vi "pulse Tx 16 spc.vi"(8 "clear DDS":bool, 9 "enable line":bool=TRUE, 10 "take it!":bool, 11 "Cluster":T2={"PW"=0, "frequency shift"=0.0, "amp"=0.9999923706054688, "mode type"=enum."CW", "mode depth"=0, "mode filter"=0, "phase shift"=0.0, "pulse shape filter"=0}) -> (0 "output valid":bool, 1 "IQ out":T1[](array[typedef]), 2 "free dds":bool, 4 "frequncy":fxp<+/-,48,0>, 6 "phase":fxp<+/-,16,1>)   [LabVIEW 2021]
uses:
  pulse_tx_vis/pdw.ctl
  pulse_tx_vis/CTL/mode_type.ctl
  <instrlib>/_niInstr/DSP/v1/Shared/Public/IQ Data.ctl
  <instrlib>/_niInstr/DSP/v1/FPGA/Public/Sub VIs/Frequency Shift/Frequency Shift - 16 spc.vi
  <instrlib>/_niInstr/Basic Elements/v1/FPGA/Private/Count Up U32.vi
  <vilib>/rvi/FXPMathLib/FxpAdd/XNode/nifxpmath_Add.xnode
  <instrlib>/_niInstr/DSP/v1/Shared/niInstr DSP v1 Shared.lvlib
  <instrlib>/_niInstr/Basic Elements/v1/FPGA/niInstr Basic Elements v1 FPGA.lvlib
  <vilib>/rvi/FXPMathLib/sim/FxpSim.dll
  <instrlib>/_niInstr/DSP/v1/FPGA/niInstr DSP v1 FPGA.lvlib
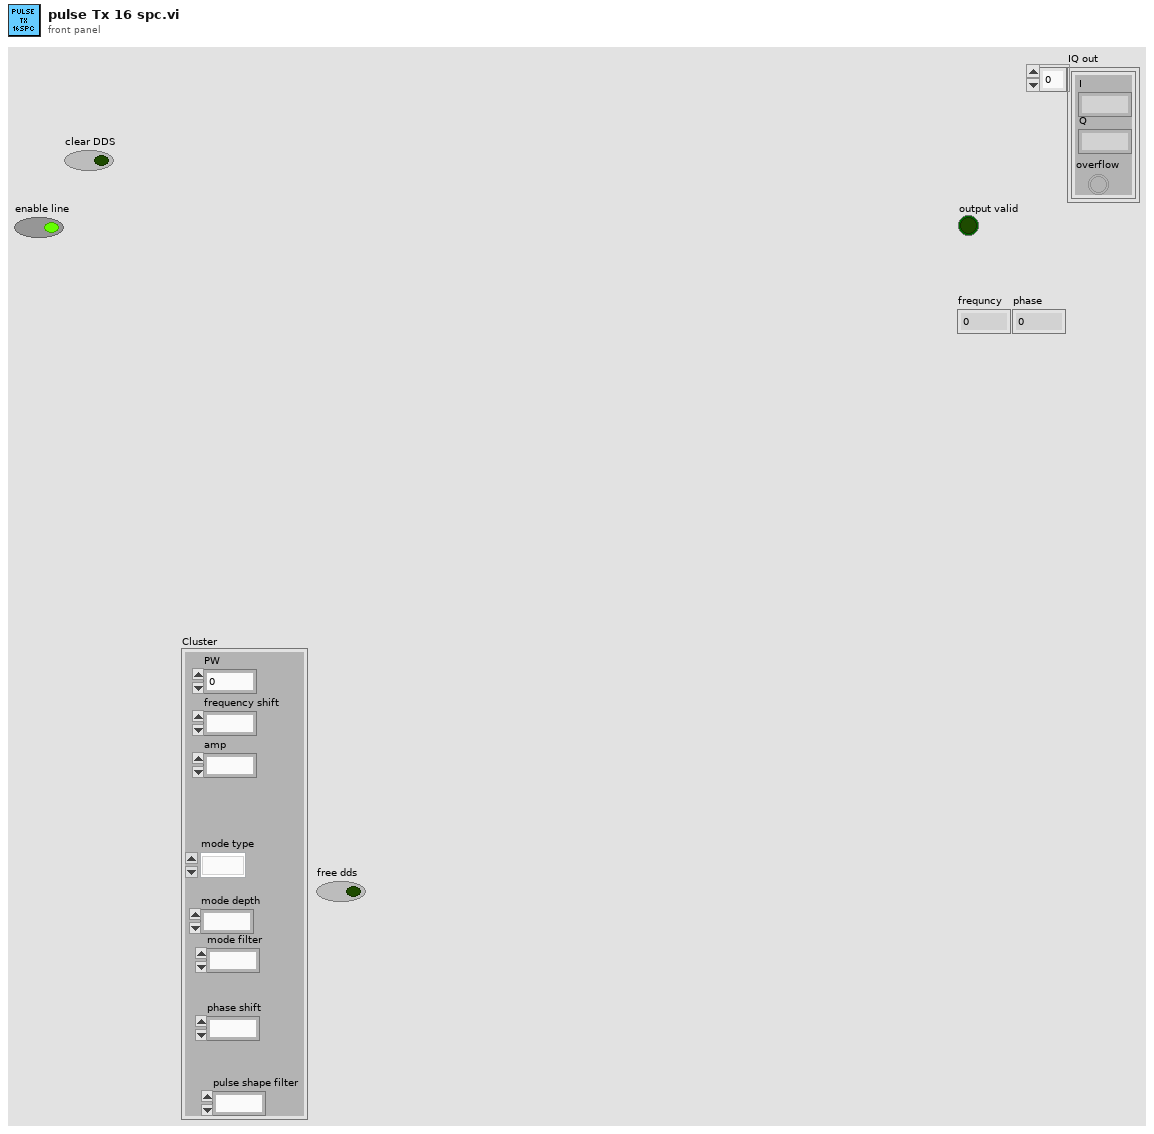
[diagram p1: front panel]
types:
  T1 = typedef "niInstr DSP v1 Shared.lvlib/IQ Data.ctl" = cluster{"I":fxp<+/-,18,1>, "Q":fxp<+/-,18,1>, "overflow":bool}
  T2 = typedef "pdw.ctl" = cluster{"PW":u32, "frequency shift":fxp<+/-,48,0>, "amp":fxp<+/-,18,1>, "mode type":T3, "mode depth":u32, "mode filter":u8, "phase shift":fxp<+/-,16,1>, "pulse shape filter":u8}
  T3 = typedef "mode_type.ctl" = enum8{"CW", "from memory 1", "NC - cw", "LFM", "BPSK", "QPSK"}
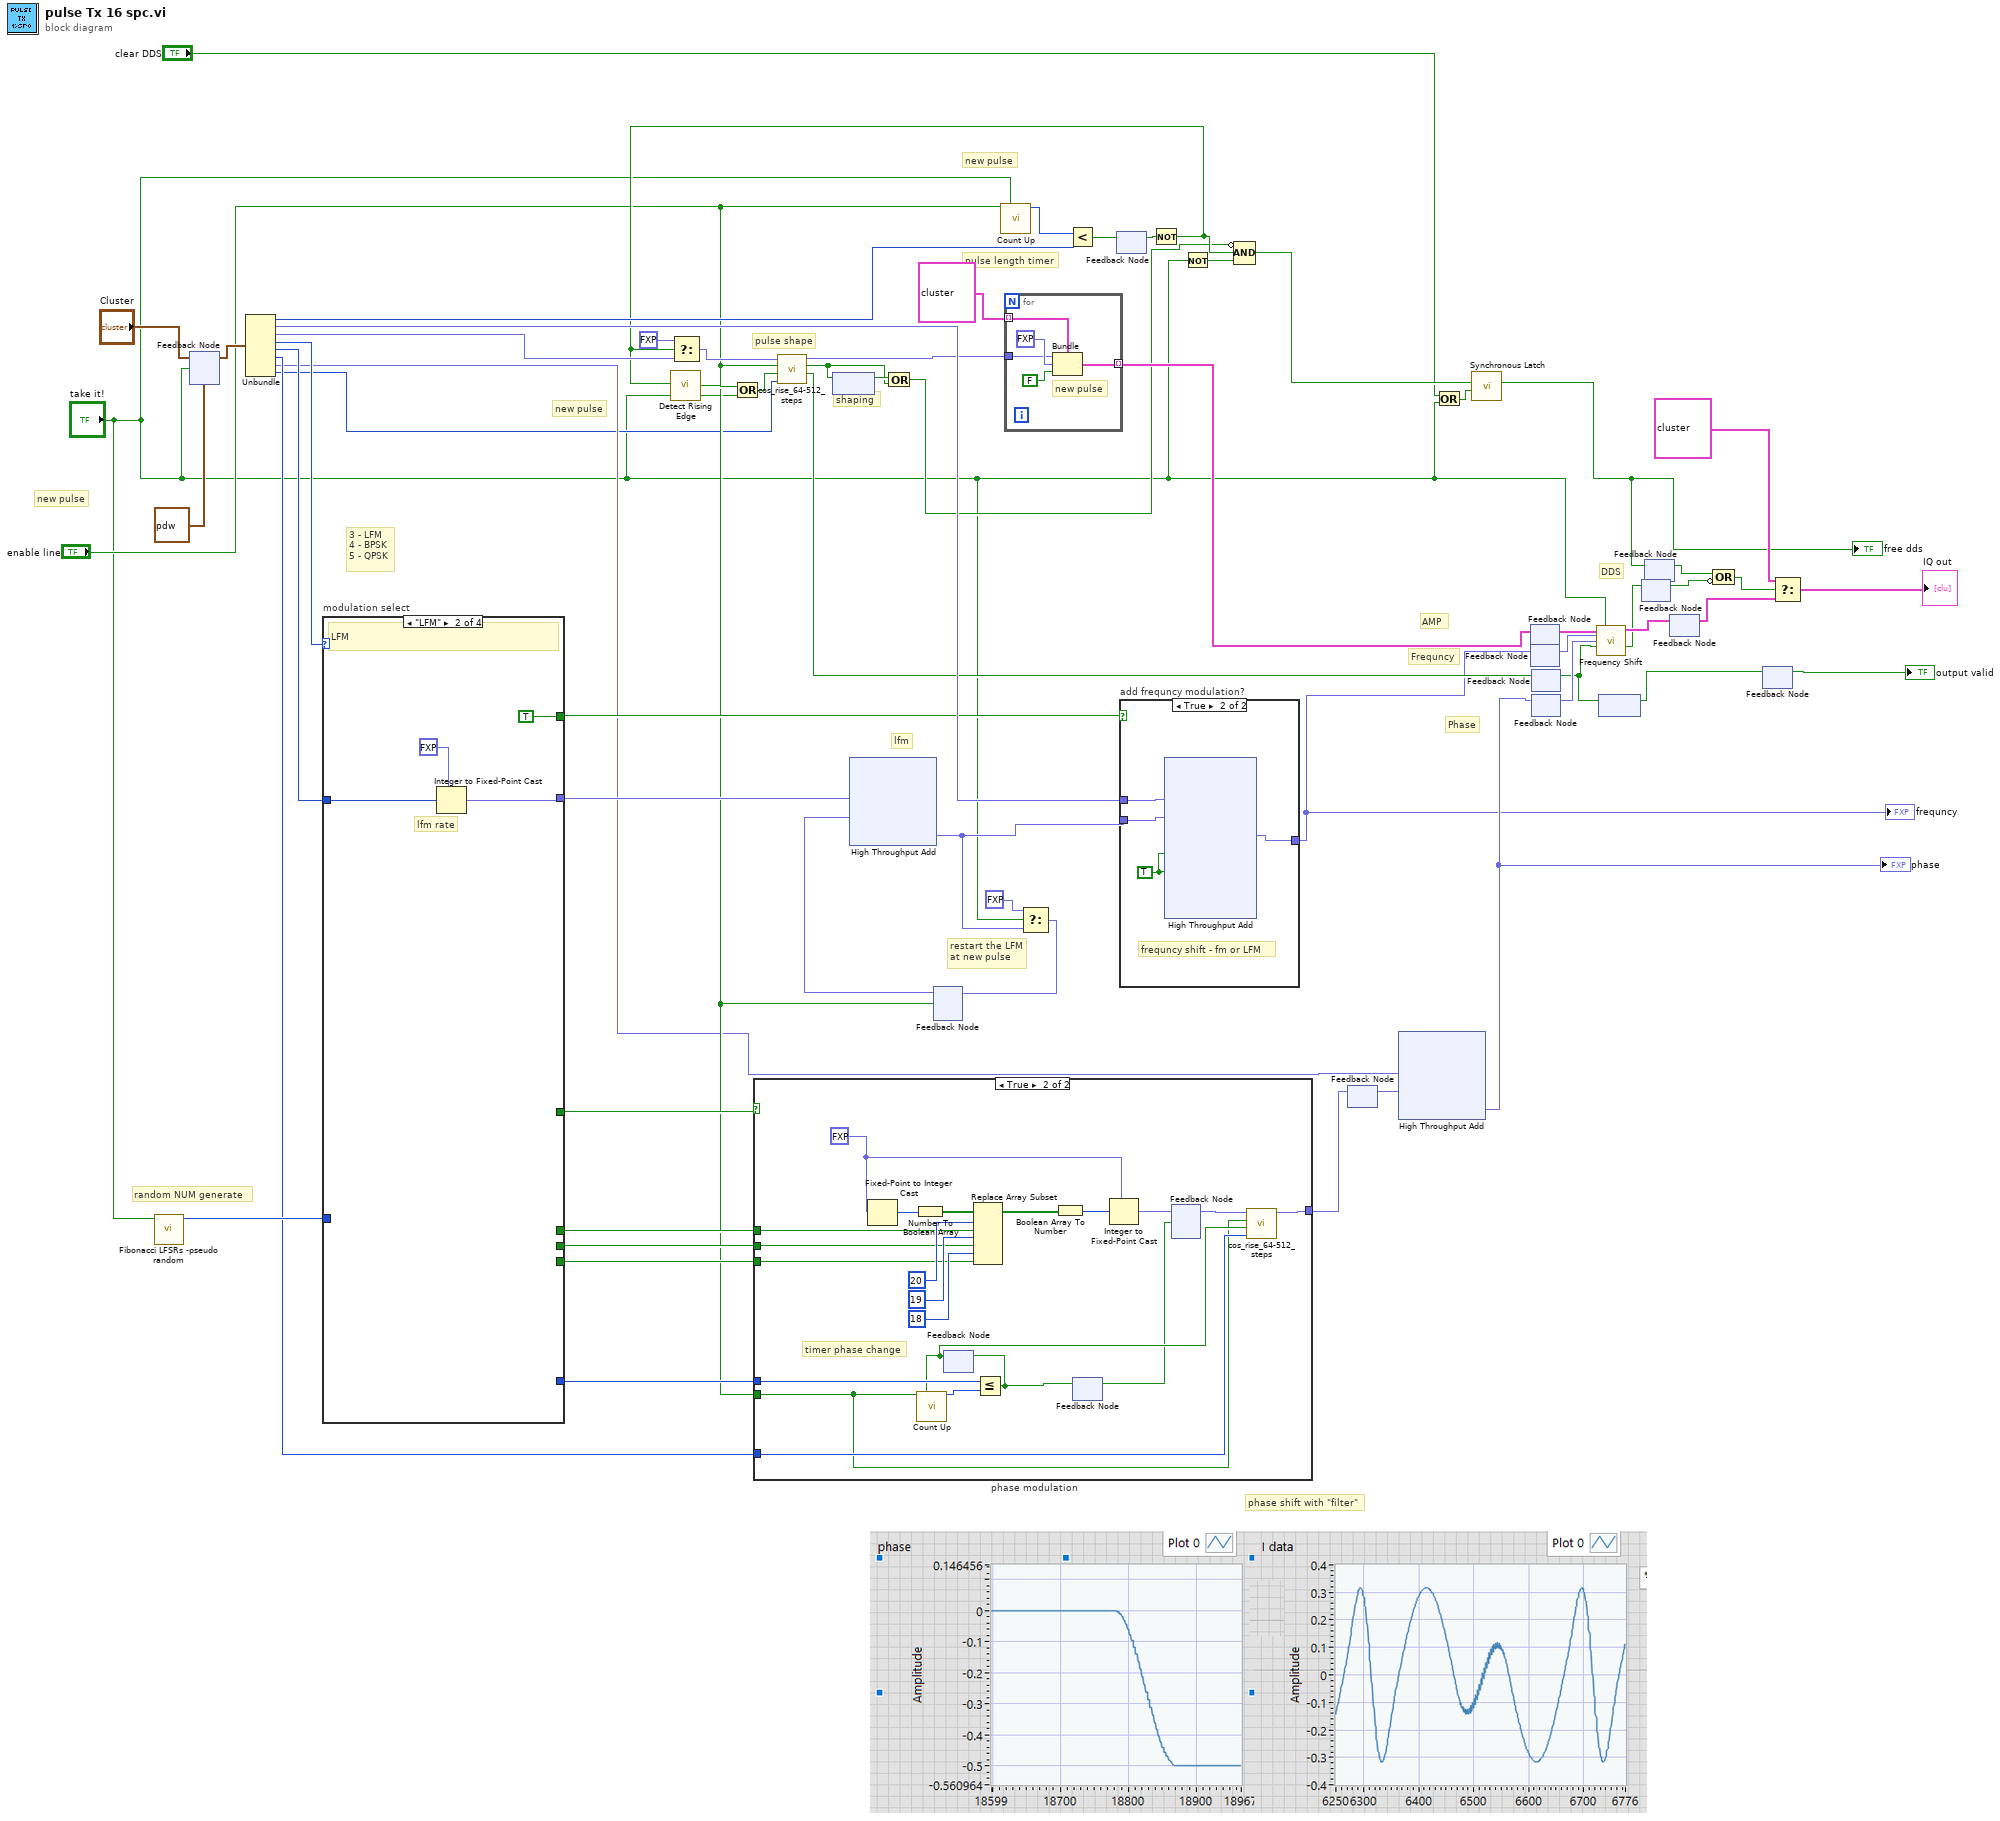
[diagram p0: block diagram]
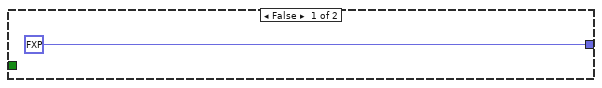
[diagram p2: hidden frame]
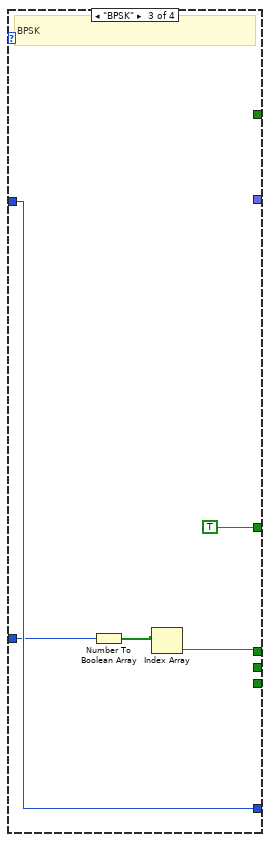
[diagram p5: hidden frame]
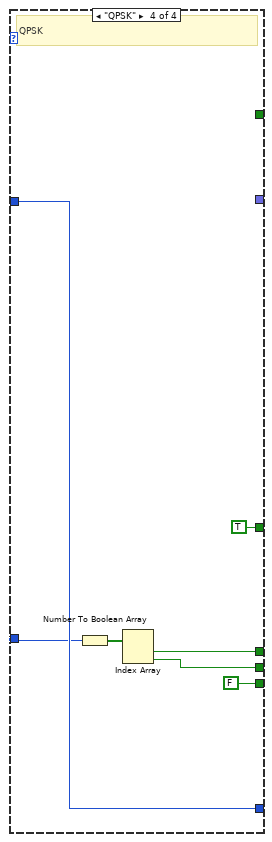
[diagram p6: hidden frame]
diagram:
  # "random NUM generate"
  # "phase shift with \"filter\""
  # "Phase"
  # "Frequncy"
  # "AMP"
  # "DDS"
  # "shaping"
  # "3 - LFM\n4 - BPSK\n5 - QPSK"
  # "pulse length timer"
  # "restart the LFM\nat new pulse"
  # "lfm"
  # "pulse shape"
  # "new pulse"
  # "new pulse"
  # "new pulse"
  n1 = call "Fibonacci LFSRs -pseudo random.vi"("reset random"="take it!") -> ("rand number"=w38:u16)  [unwired: 10 in]
  n2 = feedback #1(T2 {"PW"=0, "frequency shift"=0.0, "amp"=0.9999923706054688, "mode type"=enum."CW", "mode depth"=0, "mode filter"=0, "phase shift"=0.0, "pulse shape filter"=0} ("Cluster")) -> (w61:T2)
  n3 = feedback-in #1("Cluster", "take it!") -> ()
  n4 = Unbundle(w61) -> ("PW"=w63:u32, "frequency shift"=w57:fxp<+/-,48,0>, "amp"=w41:fxp<+/-,18,1>, "mode type"=w58:T3, "mode depth"=w33:u32, "mode filter"=w32:u8, "phase shift"=w30:fxp<+/-,16,1>, "pulse shape filter"=w16:u8)
  n5 = case "modulation select" shown="\"LFM\"" w58 {
    tunnel: w33 -> [_ w66 w69 w74]
    tunnel: [_ w65 _ _] -> w54
    tunnel: [_ TRUE ("s") _ _] -> w51
    tunnel: [_ _ _ FALSE] -> w49
    tunnel: [_ _ _ w76] -> w48
    tunnel: [_ _ w71 w78] -> w47
    tunnel: [_ _ TRUE TRUE] -> w46
    tunnel: [_ _ w69 w74] -> w45
    tunnel: w38 -> [_ _ w68 w73]
    frame Default {
    }
    frame "LFM" {
      # "lfm rate"
      # "LFM"
      n6 = Integer to Fixed-Point Cast(fixed-point type=fxp<+,32,-16> 0.0, integer=w66) -> (fixed-point=w65:fxp<+,32,-16>)
    }
    frame "BPSK" {
      # "BPSK"
      n7 = Number To Boolean Array(number=w68) -> (Boolean array=w72:bool[])
      n8 = Index Array(array=w72) -> (element=w71:bool)  [unwired: 1 in]
    }
    frame "QPSK" {
      # "QPSK"
      n9 = Number To Boolean Array(number=w73) -> (Boolean array=w79:bool[])
      n10 = Index Array(array=w79) -> (element #1=w78:bool, element #2=w76:bool)  [unwired: 2 in]
    }
  }
  n11 = case "phase modulation" shown="True" w46 {
    tunnel: w49 -> [_ w93]
    tunnel: w48 -> [_ w92]
    tunnel: w47 -> [_ w91]
    tunnel: w45 -> [_ w89]
    tunnel: [fxp<+/-,16,1> 0.0 ("filter out") w86] -> w18
    tunnel: w32 -> [_ w84]
    tunnel: "enable line" -> [_ w83]
    frame False {
    }
    frame True {
      w95 = fxp<+/-,21,0> 0.0 ("phase")
      # "timer phase change"
      n12 = Fixed-Point to Integer Cast(1:w95) -> (0:w101:i32)
      n13 = Number To Boolean Array(number=w101) -> (Boolean array=w99:bool[])
      n14 = feedback #2() -> (w85:bool)  [unwired: 1 in]
      n15 = call-poly <instrlib>:"Count Up.vi"("increment"=w83, "reset"=w85) -> ("count out"=w88:u32)  [unwired: 13 in]
      n16 = Replace Array Subset(array=w99, new element #1=w91, index #1=20 ("index"), new element #2=w92, index #2=19 ("index"), new element #3=w93, index #3=18 ("index")) -> (w94:bool[])
      n17 = Less Or Equal?(x=w89, y=w88) -> (x <= y?=w82:bool)
      n18 = feedback-in #2(w82) -> ()
      n19 = Boolean Array To Number(Boolean array=w94) -> (number=w100:u32)
      n20 = feedback-in #3(w82) -> ()
      n21 = feedback #3() -> (w81:bool)  [unwired: 1 in]
      n22 = Integer to Fixed-Point Cast(fixed-point type=w95, integer=w100) -> (fixed-point=w90:fxp<+/-,21,0>)
      n23 = feedback-in #4(w90, w81) -> ()
      n24 = feedback #4() -> (w87:fxp<+/-,21,0>)  [unwired: 1 in]
      n25 = call "cos_rise_64-512_steps.vi"("filter select"=w84, "new step"=w85, "run"=w83, "data in"=w87) -> ("data out"=w86:fxp<+/-,16,1>)  [unwired: 5 in, 2 out]
    }
  }
  n26 = feedback #5() -> (w6:bool)  [unwired: 1 in]
  n27 = feedback #6() -> (w53:fxp<+/-,48,0>)  [unwired: 1 in]
  n28 = xnode ("High Throughput Add")("x"=w54, "y"=w53) -> ("x+y"=w52:fxp<+/-,48,0>)
  n29 = call-poly <instrlib>:"Count Up.vi"("increment"="enable line", "reset"="take it!") -> ("count out"=w44:u32)  [unwired: 13 in]
  n30 = Select(t=fxp<+/-,48,0> 0.0, s="take it!", f=w52) -> (s? t:f=w55:fxp<+/-,48,0>)
  n31 = feedback-in #6(w55, "enable line") -> ()
  n32 = Less?(x=w44, y=w63) -> (x < y?=w43:bool)
  n33 = feedback #7() -> (w42:bool)  [unwired: 1 in]
  n34 = feedback-in #7(w43) -> ()
  n35 = case "add frequncy modulation?" shown="True" w51 {
    tunnel: w57 -> [w102 w106]
    tunnel: w52 -> [_ w105]
    tunnel: [w102 w104] -> w27
    frame False {
    }
    frame True {
      w103 = TRUE ("input valid")
      # "frequncy shift - fm or LFM"
      n36 = xnode ("High Throughput Add")("x"=w106, "y"=w105, "input valid"=w103, "ready for output (T)"=w103) -> ("x+y"=w104:fxp<+/-,48,0>)  [unwired: 2 out]
    }
  }
  "frequncy" <- w27
  n37 = Not(x=w42) -> (.not. x?=w35:bool)
  n38 = call <instrlib>:"Detect Rising Edge.vi"("signal"=w35) -> ("edge detected"=w34:bool)  [unwired: 14 in]
  n39 = Select(t=fxp<+/-,18,1> 0.0, s=w35, f=w41) -> (s? t:f=w40:fxp<+/-,18,1>)
  n40 = Or(x=w34, y="take it!") -> (x .or. y?=w36:bool)
  n41 = call "cos_rise_64-512_steps.vi"("filter select"=w16, "new step"=w36, "run"="enable line", "data in"=w40) -> ("output valid"=w28:bool, "steping"=w5:bool, "data out"=w37:fxp<+/-,16,1>)  [unwired: 5 in]
  n42 = feedback-in #5(w5) -> ()
  n43 = Or(x=w6, y=w5) -> (x .or. y?=w4:bool)
  n44 = for {
    tunnel: w37 -> [w109]
    tunnel: [w108] -> w26 mode=indexing
    tunnel: T1[] [{"I"=0.0, "Q"=0.0, "overflow"=FALSE}, {"I"=0.0, "Q"=0.0, "overflow"=FALSE}, {"I"=0.0, "Q"=0.0, "overflow"=FALSE}, {"I"=0.0, "Q"=0.0, "overflow"=FALSE}, {"I"=0.0, "Q"=0.0, "overflow"=FALSE}, {"I"=0.0, "Q"=0.0, "overflow"=FALSE}, {"I"=0.0, "Q"=0.0, "overflow"=FALSE}, {"I"=0.0, "Q"=0.0, "overflow"=FALSE}, {"I"=0.0, "Q"=0.0, "overflow"=FALSE}, {"I"=0.0, "Q"=0.0, "overflow"=FALSE}, {"I"=0.0, "Q"=0.0, "overflow"=FALSE}, {"I"=0.0, "Q"=0.0, "overflow"=FALSE}, {"I"=0.0, "Q"=0.0, "overflow"=FALSE}, {"I"=0.0, "Q"=0.0, "overflow"=FALSE}, {"I"=0.0, "Q"=0.0, "overflow"=FALSE}, {"I"=0.0, "Q"=0.0, "overflow"=FALSE}] ("t") -> [w107] mode=indexing
    # "new pulse"
    n45 = Bundle(cluster=w107, "I"=w109, "Q"=fxp<+/-,18,1> 0.0, "overflow"=FALSE ("input valid")) -> (w108:T1)
  }
  n46 = Not(x="take it!") -> (.not. x?=w60:bool)
  n47 = Compound Arithmetic op=AND(invert w4, w35, w60) -> (w59:bool)
  n48 = feedback-in #8(w18) -> ()
  n49 = feedback #8() -> (w17:fxp<+/-,16,1>)  [unwired: 1 in]
  n50 = xnode ("High Throughput Add")("x"=w30, "y"=w17) -> ("x+y"=w29:fxp<+/-,16,1>)
  "phase" <- w29
  n51 = Or(x="clear DDS", y="take it!") -> (x .or. y?=w1:bool)
  n52 = call <instrlib>:"Synchronous Latch.vi"("clear"=w1, "set"=w59) -> ("out"=w8:bool)  [unwired: 9 in]
  "free dds" <- w8
  n53 = feedback #9() -> (w21:T1[])  [unwired: 1 in]
  n54 = feedback-in #9(w26) -> ()
  n55 = feedback #10() -> (w25:fxp<+/-,48,0>)  [unwired: 1 in]
  n56 = feedback-in #10(w27) -> ()
  n57 = feedback #11() -> (w13:bool)  [unwired: 1 in]
  n58 = feedback-in #11(w28) -> ()
  n59 = feedback-in #12(w29) -> ()
  n60 = feedback #12() -> (w24:fxp<+/-,16,1>)  [unwired: 1 in]
  n61 = call-poly <instrlib>:"Frequency Shift.vi"("data in"=w21, "reset"="take it!", "frequency shift"=w25, "phase"=w24, "input valid"=w13) -> ("data out"=w20:T1[], "output valid"=w10:bool)  [unwired: 7 in, 2 out]
  n62 = feedback #13() -> (w12:bool)  [unwired: 1 in]
  n63 = feedback-in #13(w13) -> ()
  n64 = feedback #14() -> (w9:bool)  [unwired: 1 in]
  n65 = feedback-in #14(w10) -> ()
  n66 = feedback #15() -> (w7:bool)  [unwired: 1 in]
  n67 = feedback-in #15(w8) -> ()
  n68 = feedback #16() -> (w19:T1[])  [unwired: 1 in]
  n69 = feedback-in #16(w20) -> ()
  n70 = Compound Arithmetic op=OR(w7, invert w9) -> (w15:bool)
  n71 = feedback #17() -> (→"output valid":bool)  [unwired: 1 in]
  n72 = feedback-in #17(w12) -> ()
  n73 = Select(t=T1[] [{"I"=0.0, "Q"=0.0, "overflow"=FALSE}, {"I"=0.0, "Q"=0.0, "overflow"=FALSE}, {"I"=0.0, "Q"=0.0, "overflow"=FALSE}, {"I"=0.0, "Q"=0.0, "overflow"=FALSE}, {"I"=0.0, "Q"=0.0, "overflow"=FALSE}, {"I"=0.0, "Q"=0.0, "overflow"=FALSE}, {"I"=0.0, "Q"=0.0, "overflow"=FALSE}, {"I"=0.0, "Q"=0.0, "overflow"=FALSE}, {"I"=0.0, "Q"=0.0, "overflow"=FALSE}, {"I"=0.0, "Q"=0.0, "overflow"=FALSE}, {"I"=0.0, "Q"=0.0, "overflow"=FALSE}, {"I"=0.0, "Q"=0.0, "overflow"=FALSE}, {"I"=0.0, "Q"=0.0, "overflow"=FALSE}, {"I"=0.0, "Q"=0.0, "overflow"=FALSE}, {"I"=0.0, "Q"=0.0, "overflow"=FALSE}, {"I"=0.0, "Q"=0.0, "overflow"=FALSE}], s=w15, f=w19) -> (s? t:f=→"IQ out":T1[])
